vi "Half Speed Converter.vi"(2 "Enable":bool, 3 "Y axis":dbl, 4 "X axis":dbl) -> (0 "Y axis":dbl, 1 "X axis":dbl)   [LabVIEW 2013]
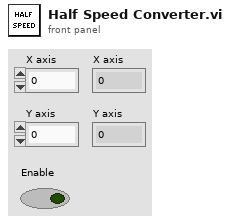
[diagram p1: front panel]
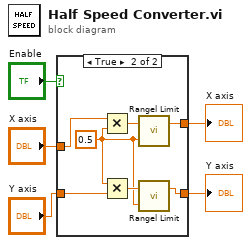
[diagram p0: block diagram]
diagram:
  n1 = case shown="True" "Enable" {
    tunnel: "X axis" -> [w7 w14]
    tunnel: "Y axis" -> [w6 w13]
    tunnel: [w6 w8] -> w3
    tunnel: [w7 w11] -> w2
    frame False {
    }
    frame True {
      w9 = 0.5 ("x")
      n2 = Multiply(x=w14, y=w9) -> (x*y=w12:dbl)
      n3 = Multiply(x=w9, y=w13) -> (x*y=w10:dbl)
      n4 = call "Rangel Limit.vi"("Limit"=w9, "Input"=w12) -> ("Output"=w11:dbl)  [unwired: 1 in]
      n5 = call "Rangel Limit.vi"("Limit"=w9, "Input"=w10) -> ("Output"=w8:dbl)  [unwired: 1 in]
    }
  }
  "X axis" <- w2
  "Y axis" <- w3
